vi "Adv_ReadLightFieldProperty.vi"(8 "error in (no error)":errorcluster, 10 "setting":string, 11 "LightField Automation in":refnum<class "LightField Automation.lvclass">) -> (0 "error out":errorcluster, 2 "value":refnum<k24>, 3 "LightField Automation out":refnum<class "LightField Automation.lvclass">)   [LabVIEW 2013, in "LightField Automation.lvclass"]
uses:
  LightField Automation.lvclass
  LightField Automation.lvclass/LightField Automation.ctl
  C:/Program Files/Princeton Instruments/LightField/AddInViews/PrincetonInstruments.LightFieldViewV3.dll
  Program Files/Princeton Instruments/LightField/AddInViews/PrincetonInstruments.LightFieldViewV3.dll
  <vilib>/Utility/error.llb/DialogType.ctl
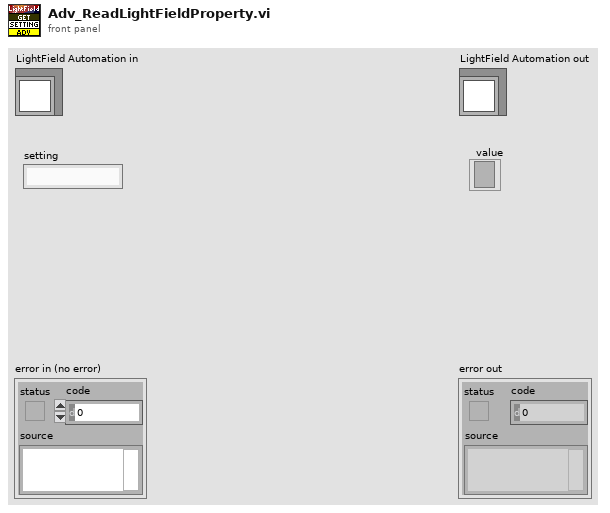
[diagram p1: front panel]
types:
  T1 = typedef "DialogType.ctl" = u16
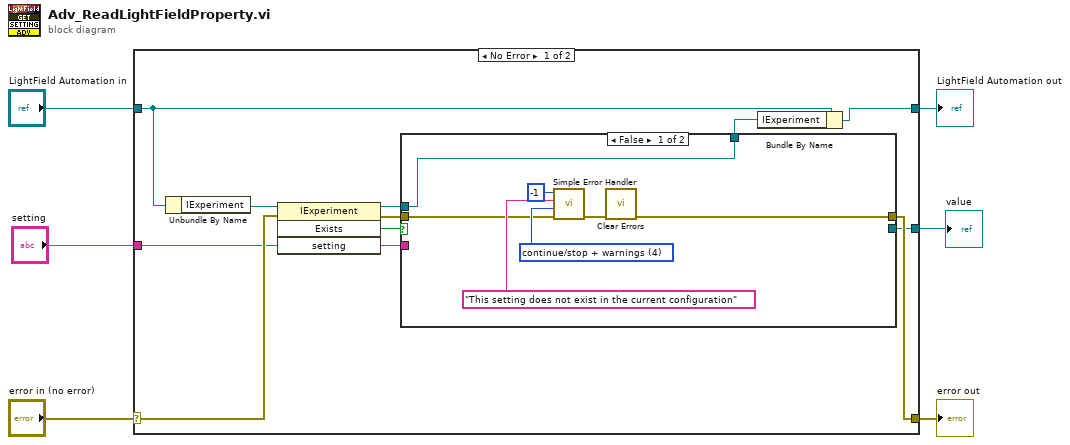
[diagram p0: block diagram]
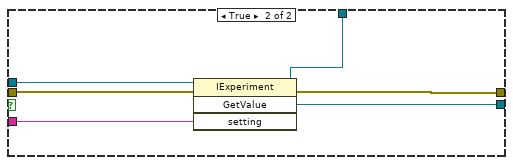
[diagram p2: hidden frame]
diagram:
  n1 = case shown="No Error" "error in (no error)" {
    selector: "error in (no error)" -> [w15 w32]
    tunnel: [w17 w32] -> w5
    tunnel: [w8 w31] -> w3
    tunnel: "LightField Automation in" -> [w9 w31]
    tunnel: "setting" -> [w11 _]
    tunnel: [w10 _] -> w1
    frame No Error {
      n2 = Unbundle By Name(w9) -> ("IExperiment"=w16:refnum<k24>)
      n3 = invoke class="IExperiment" method="Exists"(reference=w16, error in=w15, "setting"=w11) -> (reference out=w13:refnum<k24>, error out=w12:errorcluster, "Exists"=w14:bool)  [unwired: 1 in, 1 out]
      n4 = case shown="False" w14 {
        tunnel: [w21 w25] -> w17
        tunnel: w13 -> [w18 w30]
        tunnel: w12 -> [w19 w29]
        tunnel: w11 -> [_ w28]
        tunnel: [_ w27] -> w10
        tunnel: [w18 w26] -> w7
        frame False {
          w20 = T1 4 items=["no dialog", "OK message", "continue or stop message", "OK message + warnings", "continue/stop + warnings"] ("type of dialog (OK msg:1)")
          n5 = call <vilib>:"Simple Error Handler.vi"("error code (no error:0)"=-1, "error source (\" \")"="This setting does not exist in the current configuration" ("source"), "type of dialog (OK msg:1)"=w20, "error in (no error)"=w19) -> ("error out"=w22:errorcluster)  [unwired: 1 in, 4 out]
          n6 = call <vilib>:"Clear Errors.vi"("error in (no error)"=w22) -> ("error out"=w21:errorcluster)  [unwired: 6 in]
        }
        frame True {
          n7 = invoke class="IExperiment" method="GetValue"(reference=w30, error in=w29, "setting"=w28) -> (reference out=w26:refnum<k24>, error out=w25:errorcluster, "GetValue"=w27:refnum<k24>)  [unwired: 1 in, 1 out]
        }
      }
      n8 = Bundle By Name(cluster=w9, "IExperiment"=w7) -> (w8:refnum<class "LightField Automation.lvclass">)
    }
    frame Error {
    }
  }
  "error out" <- w5
  "LightField Automation out" <- w3
  "value" <- w1
